vi "Connect.vi"(8 "error in (no error)":errorcluster, 9 "Serial Config":T1 {"Parity" items=["None", "Odd", "Even"]; "Flow Ctl" items=["None"]; "Baud" items=["4800"=4800, "9600"=9600, "19200"=19200, "38400"=38400]}, 10 "VISA resource name":refnum<visa-resource-name>, 11 "B&K Precision 9120 series in":refnum<class "B&K Precision 9120 series.lvclass">) -> (0 "error out":errorcluster, 1 "result":string, 3 "B&K Precision 9120 series out":refnum<class "B&K Precision 9120 series.lvclass">)   [LabVIEW 2014, in "B&K Precision 9120 series.lvclass"]
uses:
  B&K Precision 9120 series.lvclass
  Serial_Config.ctl
  B&K Precision 9120 series.lvclass/B&K Precision 9120 series.ctl
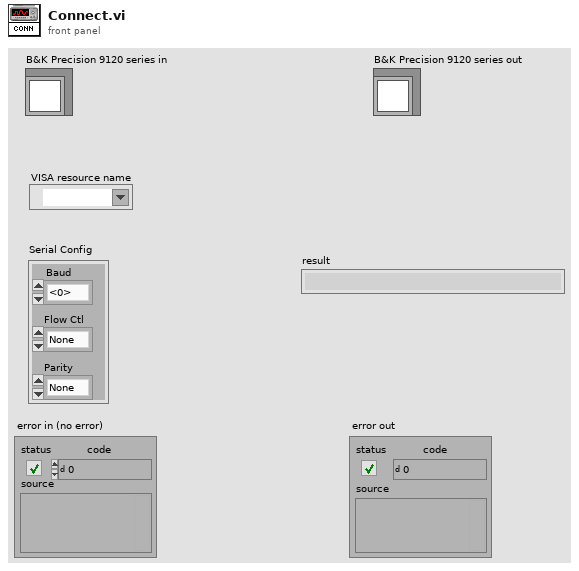
[diagram p1: front panel]
types:
  T1 = typedef "B&K Precision 9120 series.lvclass/Serial_Config.ctl" = cluster{"Baud":u32, "Flow Ctl":u16, "Parity":u16}
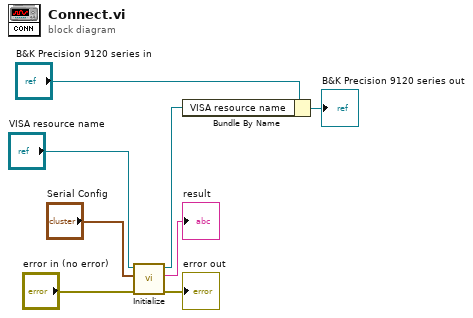
[diagram p0: block diagram]
diagram:
  n1 = call "Initialize.vi"("error in (no error)"="error in (no error)", "Serial Config"="Serial Config", "VISA resource in"="VISA resource name") -> ("error out"=→"error out":errorcluster, "read buffer"=→"result":string, "VISA resource out"=w2:refnum<visa-resource-name>)  [unwired: 6 in]
  n2 = Bundle By Name(cluster="B&K Precision 9120 series in", "VISA resource name"=w2) -> (→"B&K Precision 9120 series out":refnum<class "B&K Precision 9120 series.lvclass">)
